vi "IB_RW_Project_RegData_I32.vi"(7 "action":T3, 8 "error in (no error)":errorcluster, 9 "index in":string, 10 "RegData":T2, 11 "buildObject":T1) -> (0 "error out":errorcluster, 1 "index out":string, 2 "RegData":T2, 3 "buildObject out":T1)   [LabVIEW 2020]
doc: "Reads and writes the data to the object property bag."
uses:
  <resource>/Framework/Providers/API/ItemRef.ctl
  <vilib>/AppBuilder/IB_RW_Project/IB_RW_Project_RegData_I32_Data.ctl
  <vilib>/AppBuilder/IB_RW_Project/IB_RW_Project_PropBag_Action.ctl
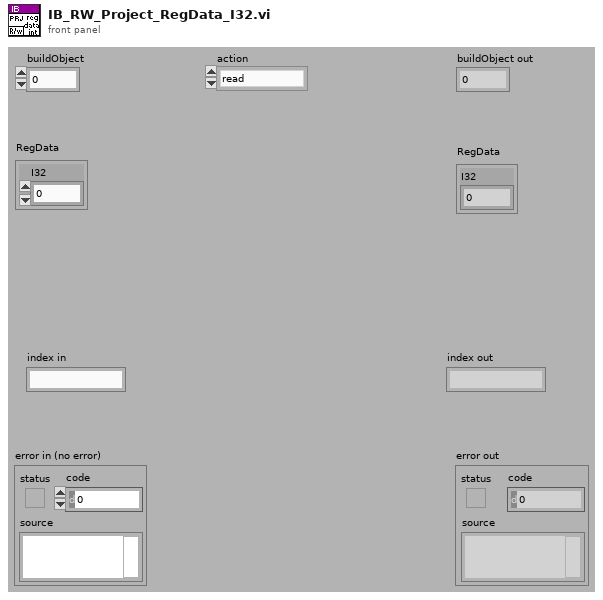
[diagram p1: front panel]
types:
  T1 = typedef "ItemRef.ctl" = u64
  T2 = typedef "IB_RW_Project_RegData_I32_Data.ctl" = cluster{"I32":i32}
  T3 = typedef "IB_RW_Project_PropBag_Action.ctl" = enum16{"read", "write", "clear", "readPrevious", "writePrevious", "clearPrevious"}
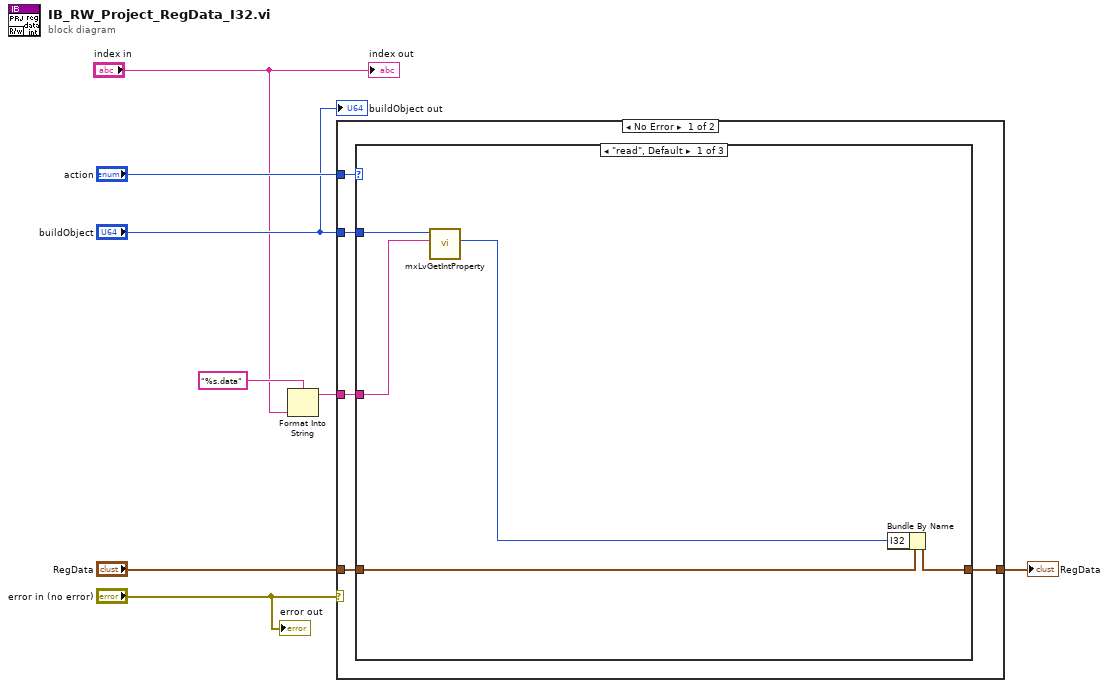
[diagram p0: block diagram]
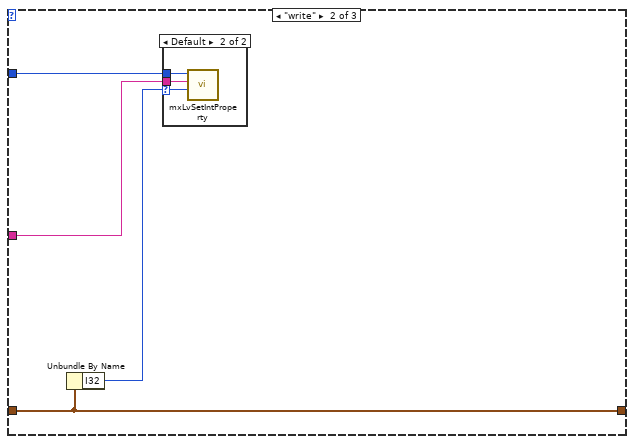
[diagram p2: hidden frame]
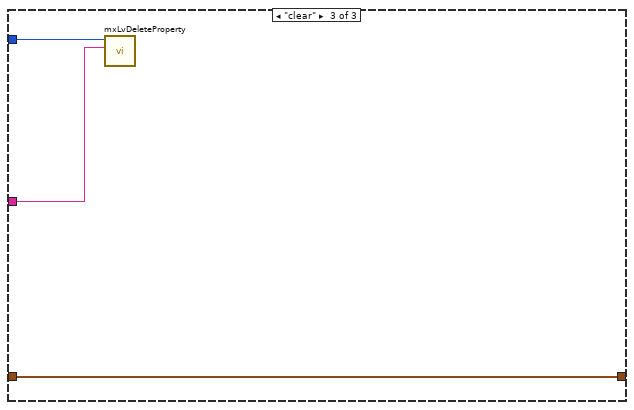
[diagram p4: hidden frame]
diagram:
  n1 = Format Into String(format string="%s.data", "index in") -> (resulting string=w5:string)  [unwired: 2 in, 1 out]
  n2 = case shown="No Error" "error in (no error)" {
    tunnel: "action" -> [w13 _]
    tunnel: "RegData" -> [w12 w29]
    tunnel: w5 -> [w11 _]
    tunnel: [w10 w29] -> w4
    tunnel: "buildObject" -> [w9 _]
    frame No Error {
      n3 = case shown="\"read\", Default" w13 {
        tunnel: w9 -> [w16 w19 w27]
        tunnel: w12 -> [w18 w22 w28]
        tunnel: w11 -> [w15 w21 w26]
        tunnel: [w17 w22 w28] -> w10
        frame "read", Default {
          n4 = call <resource>:"mxLvGetIntProperty.vi"("Tag"=w15, "Item"=w16) -> ("Value"=w14:i32)  [unwired: 1 in, 8 out]
          n5 = Bundle By Name(cluster=w18, "I32"=w14) -> (w17:T2)
        }
        frame "write" {
          n6 = Unbundle By Name(w22) -> ("I32"=w20:i32)
          n7 = case shown="Default" w20 {
            selector: w20 -> [_ w24]
            tunnel: w21 -> [_ w25]
            tunnel: w19 -> [_ w23]
            frame 0 {
            }
            frame Default {
              n8 = call <resource>:"mxLvSetIntProperty.vi"("Value (0)"=w24, "Tag"=w25, "Item"=w23) -> ()  [unwired: 2 in, 7 out]
            }
          }
        }
        frame "clear" {
          n9 = call <resource>:"mxLvDeleteProperty.vi"("Tag"=w26, "Item"=w27) -> ()  [unwired: 1 in, 9 out]
        }
      }
    }
    frame Error {
    }
  }
  "RegData" <- w4
  "error out" <- "error in (no error)"
  "buildObject out" <- "buildObject"
  "index out" <- "index in"
